vi "Increment Run Count.vi"(8 "error in (no error)":errorcluster, 11 "CommandDirector in":refnum<class "CommandDirector.lvclass">) -> (0 "error out":errorcluster, 3 "CommandDirector out":refnum<class "CommandDirector.lvclass">)   [LabVIEW 2023, in "HAF.lvlib" / "CommandDirector.lvclass"]
doc: "Increments the Run Count which keeps track of how many times the Command Director has processed its Commands."
uses:
  CommandDirector.lvclass
  CommandDirector.lvclass/CommandDirector.ctl
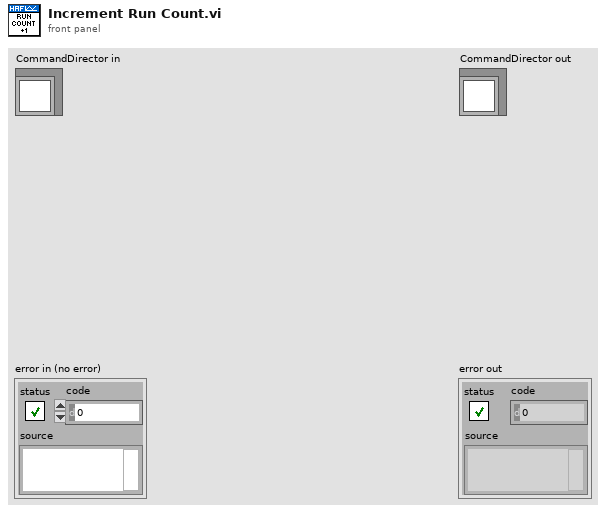
[diagram p1: front panel]
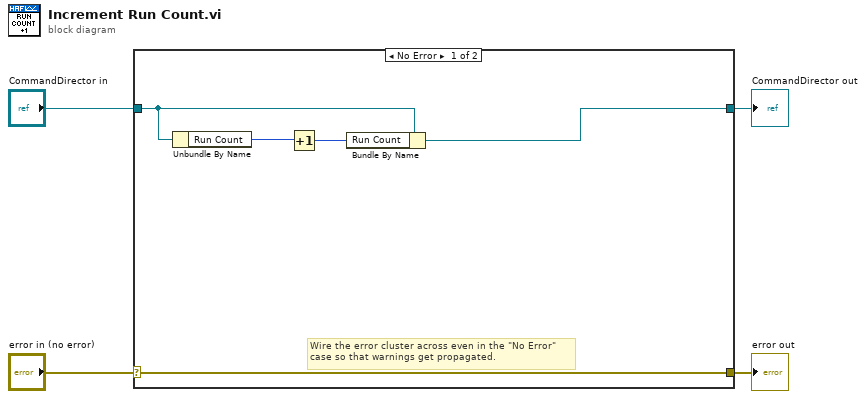
[diagram p0: block diagram]
diagram:
  n1 = case shown="No Error" "error in (no error)" {
    selector: "error in (no error)" -> [w9 w11]
    tunnel: [w9 w11] -> w3
    tunnel: [w5 w10] -> w1
    tunnel: "CommandDirector in" -> [w7 w10]
    frame No Error {
      # "Wire the error cluster across even in the \"No Error\"\ncase so that warnings get propagated."
      n2 = Unbundle By Name(w7) -> ("Run Count"=w8:u32)
      n3 = Increment(x=w8) -> (x+1=w6:u32)
      n4 = Bundle By Name(cluster=w7, "Run Count"=w6) -> (w5:refnum<class "CommandDirector.lvclass">)
    }
    frame Error {
    }
  }
  "error out" <- w3
  "CommandDirector out" <- w1
